vi "CA_CSE1_V1e_wo_LOSV2b_Driver.vi"() -> ()   [LabVIEW 2010]
uses:
  <vilib>/addons/Simulation Interface/driversupportVIs/SIT Loop Timing Attributes.ctl
  <vilib>/addons/Simulation Interface/driversupportVIs/NI_SIT_driversupportVIs.lvlib
  <vilib>/addons/Simulation Interface/_SITServer/NI_SIT_SITServer.lvlib
panel:
  in  "Tab Control":T1(tab)
  in  "port":u16=6011
  in  "Buffer Sizes":T2={"number of signals"=50, "circular buffer size"=1000, "num data points"=100}
  in  "Stop time (sec)":dbl=-1.0 format="%.3f"
  in  "Model DLL path":path=path "C:/Documents and Settings/mcl/Desktop/User Interface CSE1/model/Simulink/CA_CSE1_V1e_wo_LOSV2b_nidll_rtw/CA_CSE1_V1e_wo_LOSV2b.*"
  in  "Start Server?":bool=TRUE
  in  "Wait for Start Command":bool=TRUE
  in  "Base Rate Period (sec) (-1: use model time step)":dbl=-1.0
  in  "Server Loop Processor (-2: Automatic)":i32=-2
  in  "Task Loops Processor (0..255)":i32 min=0 max=2555
  in  "Logging Loop Timing Attributes":T3={"Processor"=-2, "Period (ms)"=10, "Priority"=2, "Offset (ms)"=0}
  in  "Replay Loop Timing Attributes":T3={"Processor"=-2, "Period (ms)"=10, "Priority"=3, "Offset (ms)"=5}
  out "error out":errorcluster
  # "Server Control"
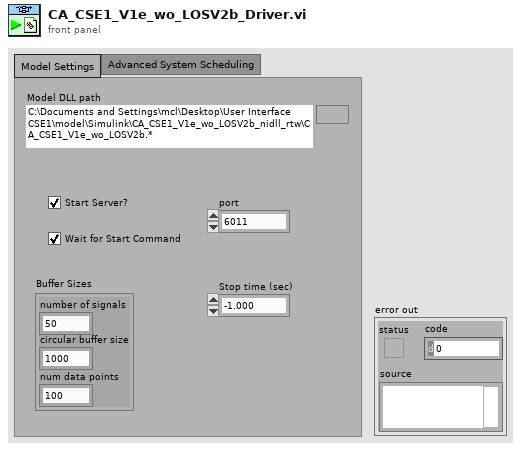
[diagram p1: front panel]
types:
  T1 = enum32{"Model Settings", "Advanced System Scheduling"}
  T2 = cluster{"number of signals":u32, "circular buffer size":u32, "num data points":u32}
  T3 = typedef "NI_SIT_driversupportVIs.lvlib/SIT Loop Timing Attributes.ctl" = cluster{"Processor":i32, "Period (ms)":i64, "Priority":i32, "Offset (ms)":i64}
  T4 = typedef "NI_SIT_driversupportVIs.lvlib/SIT Simulation Data.ctl" = cluster{"Model DLL Path":path, "model refnum":T5, "Loop Sync FIFO":refnum<k33>, "num probe signals":u32, "circular buffer size":u32, "num data points":u32, "Simulation State":refnum<k33>, "ProbeSignal FIFO":refnum<k33>, "SignalData FIFO":refnum<k33>, "SimulationCtl FIFO":refnum<k33>, "Server On?":bool, "Decimation Parameter":refnum<k33>, "Project Dir":path, "GlobalLogData":T6, "Dataloss FIFO":refnum<k33>, "TimingSrcIDs":i32[], "presized input array":dbl[], "output loop TSrcID":i32, "output loop name":string, "Outputs Ready":refnum<notifier>, "Timed Loops":string[], "GlobalReplayData":T10, "Background Loopsync":refnum<notifier>, "Set Param SemQ":refnum<queue>}
  T5 = typedef "NI_SIT_driversupportVIs.lvlib/SIT Model Refnum.ctl" = cluster{"model":i32, "number of inports":i32, "number of outports":i32, "model name":string, "number of tasks":i32, "base period (usec)":u32}
  T6 = typedef "NI_SIT_Data Log.lvlib/Global Log Data.ctl" = cluster{"Log On":bool, "Max Sizes":T7, "Cfg Comm Qs":T8, "Log Comm FIFOs":T9, "ConfigsDir":path}
  T7 = typedef "NI_SIT_Data Log.lvlib/Max Log Buffer Sizes.ctl" = cluster{"Signals":i32, "Data Pts":i32, "Groups":i32, "Total Width":i32, "Buffer Depth":i32}
  T8 = typedef "NI_SIT_Data Log.lvlib/Configuration Communication Queues.ctl" = cluster{"Log Msg Q":refnum<queue>, "Config Q":refnum<queue>}
  T9 = typedef "NI_SIT_Data Log.lvlib/Data Log Communication FIFOs.ctl" = cluster{"Packet FIFO":refnum<k33>, "Probe List FIFO":refnum<k33>}
  T10 = typedef "NI_SIT_Replay.lvlib/Global Replay Data.ctl" = cluster{"Replay On":bool, "Replay Max Sizes":T11, "FIFOs":T12, "Queues":T14, "ConfigsDir":path}
  T11 = typedef "NI_SIT_Replay.lvlib/Replay Max Sizes.ctl" = cluster{"Inports":i32, "FIFO Depth":u32}
  T12 = typedef "NI_SIT_Replay.lvlib/Replay Communication FIFOs.ctl" = cluster{"Config FIFO":refnum<k33>, "TCL Ack FIFO":refnum<k33>, "Data FIFOs":T13, "TCL Position FIFO":refnum<k33>}
  T13 = typedef "NI_SIT_Replay.lvlib/Data FIFOs.ctl" = cluster{"Data FIFO 1":refnum<k33>, "Data FIFO 2":refnum<k33>}
  T14 = typedef "NI_SIT_Replay.lvlib/Replay Queues.ctl" = cluster{"Cmd Q":refnum<queue>, "Status Queue":refnum<queue>}
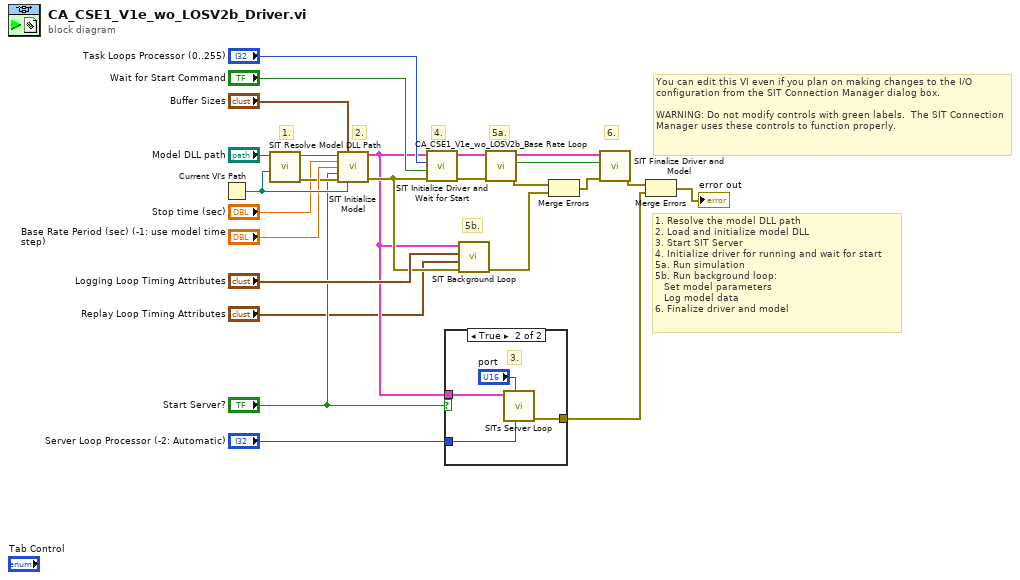
[diagram p0: block diagram]
diagram:
  # "1."
  # "You can edit this VI even if you plan on making changes to the I/O configuration from the SIT Connection Manager dialog box.\n\nWARNING: Do not modify controls with green labels.  The SIT Connection Manager uses these controls to function properly."
  # "5b."
  # "1. Resolve the model DLL path\n2. Load and initialize model DLL\n3. Start SIT Server\n4. Initialize driver for running and wait for start\n5a. Run simulation\n5b. Run background loop:\n   Set model parameters\n   Log model data\n6. Finalize driver and model"
  # "6."
  # "5a."
  # "4."
  # "2."
  n1 = Current VI's Path() -> (path=w25:path)
  n2 = call <vilib>:"SIT Resolve Model DLL Path.vi"("Driver VI Path"=w25, "Model DLL Path In"="Model DLL path") -> ("error out"=w20:errorcluster, "Resolved Model DLL Path"=w5:path)  [unwired: 1 in, 7 out]
  n3 = call <vilib>:"SIT Initialize Model.vi"("Model DLL Path"=w5, "Buffer Sizes"="Buffer Sizes", "stop time (-1: continuous)"="Stop time (sec)", "time step (sec) (-1: use model time step)"="Base Rate Period (sec) (-1: use model time step)", "Server On?"="Start Server?", "error in (no error)"=w20, "Driver VI Path"=w25) -> ("Simulation Data out"=w2:T4, "error out"=w23:errorcluster)  [unwired: 7 out]
  n4 = call <vilib>:"SIT Initialize Driver and Wait for Start.vi"("error in"=w23, "Wait for Start Command (T)"="Wait for Start Command", "Task Loops Processor (0..255)"="Task Loops Processor (0..255)", "Simulation Data in"=w2) -> ("error out"=w12:errorcluster, "Simulation Data Out"=w11:T4)  [unwired: 1 in, 5 out]
  n5 = case shown="True" "Start Server?" {
    tunnel: w2 -> [_ w29]
    tunnel: [_ w27] -> w8
    tunnel: "Server Loop Processor (-2: Automatic)" -> [_ w26]
    frame False {
    }
    frame True {
      # "3."
      n6 = call <vilib>:"SITs Server Loop.vi"("Server Loop Processor (-2: Automatic)"=w26, "port"="port", "Simulation Data in"=w29) -> ("error out"=w27:errorcluster)  [unwired: 2 in, 6 out]
    }
  }
  n7 = call <vilib>:"SIT Background Loop.vi"("error in"=w23, "Replay Loop Timing Attributes"="Replay Loop Timing Attributes", "Logging Loop Timing Attributes"="Logging Loop Timing Attributes", "Simulation Data"=w2) -> ("error out"=w10:errorcluster)  [unwired: 7 out]
  n8 = call "CA_CSE1_V1e_wo_LOSV2b_Base Rate Loop.vi"("error in (no error)"=w12, "Simulation Data"=w11) -> ("error out"=w15:errorcluster, "scheduler overrun?"=w16:bool, "Simulation Data out"=w13:T4)  [unwired: 1 in, 6 out]
  n9 = Merge Errors(w15, w10) -> (w14:errorcluster)
  n10 = call <vilib>:"SIT Finalize Driver and Model.vi"("error in"=w14, "scheduler overrun?"=w16, "Simulation Data in"=w13) -> ("error out"=w9:errorcluster)  [unwired: 1 in, 7 out]
  n11 = Merge Errors(w9, w8) -> (→"error out":errorcluster)
